vi "drive.vi"   [LabVIEW 2018]
uses:
  drive.ctl
  <vilib>/Rock Robotics/WPI/Utilities/WPI_GetSetVariantRefNum.vi
types:
  T1 = typedef "WPI_RobotDriveDevRef.ctl" = cluster{"DevStatus":errorcluster, "Motors[]":T2[], "Square Inputs":bool, "Max Output":dbl}
  T2 = typedef "WPI_MotorControlDeviceRef.ctl" = cluster{"DeviceStatus":errorcluster, "Type":T3, "PWM":cluster{"PWM Channel":T4, "DeadBand":T5}, "CAN":cluster{"Device Number":u8, "SetOutput VI Ref":variant, "GetOutput VI Ref":variant, "Enable VI Ref":variant, "Disable VI Ref":variant, "Data":variant}, "Invert":bool, "DIO PWM":cluster{"PWM \"Enable\" Channel":T4, "DIOChannel":T6, "PWM Rate":dbl}}
  T3 = typedef "WPI_MotorControlType.ctl" = enum16{"PWM", "CAN", "DIO PWM"}
  T4 = typedef "FPGA_DIOPWMChannel.ctl" = enum8{"PWM 0", "PWM 1", "PWM 2", "PWM 3", "PWM 4", "PWM 5", "PWM 6", "PWM 7", "PWM 8", "PWM 9", "PWM MXP 0", "PWM MXP 1", "PWM MXP 2", "PWM MXP 3", "PWM MXP 4", "PWM MXP 5", "PWM MXP 6", "PWM MXP 7", "PWM MXP 8", "PWM MXP 9", "Invalid"}
  T5 = typedef "WPI_PWMDeadband.ctl" = cluster{"Name":string, "maxPositivePwm":i32, "minPositivePwm":i32, "centerPwm":i32, "maxNegativePwm":i32, "minNegativePwm":i32, "angularRange":u16}
  T6 = typedef "FPGA_DIOChannel.ctl" = enum8{"DIO 0", "DIO 1", "DIO 2", "DIO 3", "DIO 4", "DIO 5", "DIO 6", "DIO 7", "DIO 8", "DIO 9", "DIO MXP 0", "DIO MXP 1", "DIO MXP 2", "DIO MXP 3", "DIO MXP 4", "DIO MXP 5", "DIO MXP 6", "DIO MXP 7", "DIO MXP 8", "DIO MXP 9", "DIO MXP 10", "DIO MXP 11", "DIO MXP 12", "DIO MXP 13", "DIO MXP 14", "DIO MXP 15", "SPI Port CS1", "SPI Port CS2", "SPI Port CS3", "SPI Port MISO", "SPI Port MOSI", "Invalid"}
  T7 = typedef "drive.ctl" = enum16{"noDrive", "Manual", "ManualWithPID"}
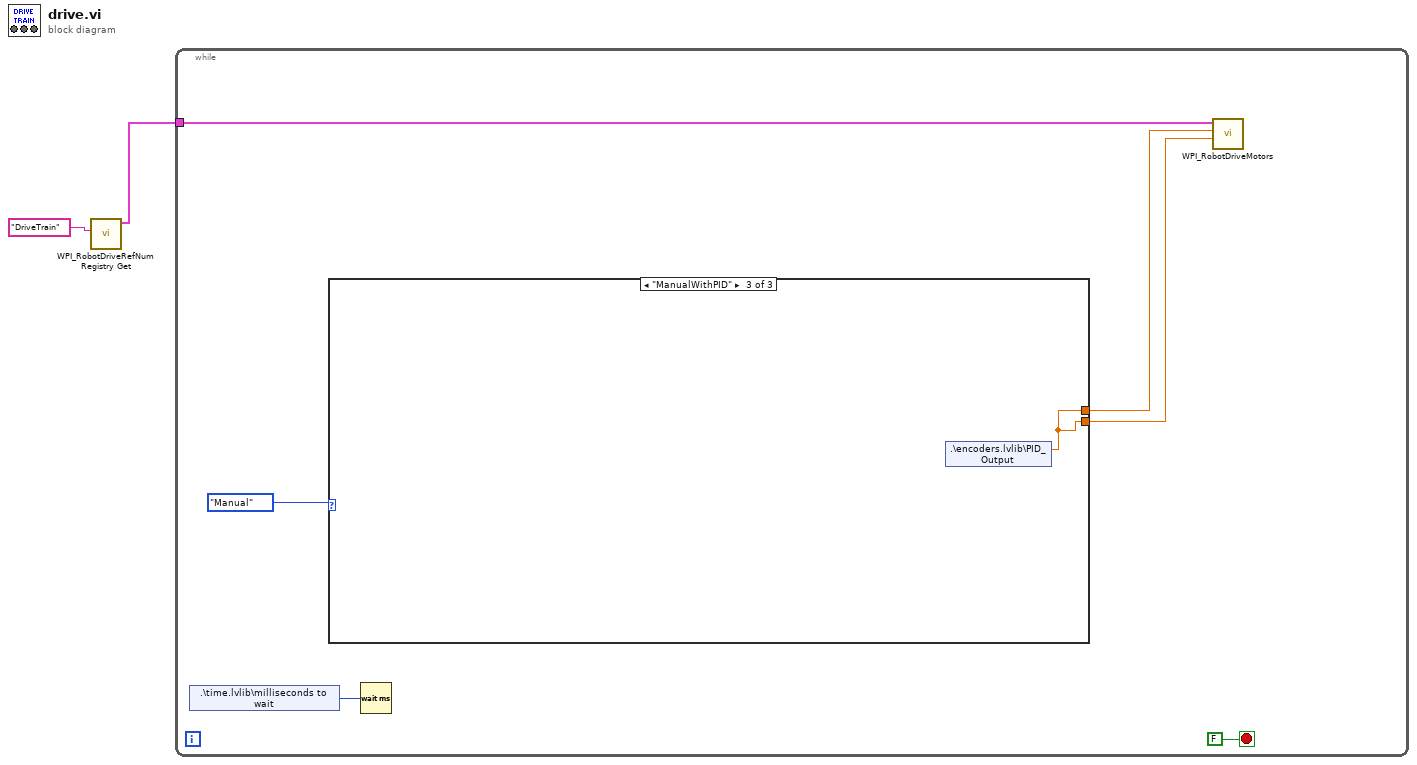
[diagram p0: block diagram]
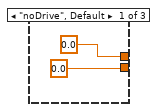
[diagram p2: hidden frame]
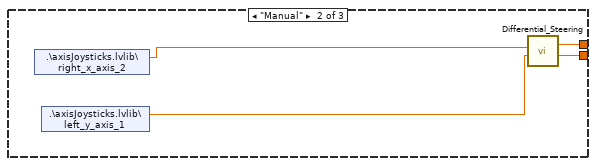
[diagram p3: hidden frame]
diagram:
  n1 = call <vilib>:"WPI_RobotDriveRefNum Registry Get.vi"("refnum name"="DriveTrain") -> ("RobotDriveDevRef"=w1:T1)  [unwired: 9 in, 1 out]
  n2 = while {
    tunnel: w1 -> [w6]
    stop <- FALSE stop-if-true
    n3 = shared-variable ".\\time.lvlib\\milliseconds to wait"() -> (w8:u32)  [unwired: 1 in, 1 out]
    n4 = case shown="\"ManualWithPID\"" drive."Manual" {
      tunnel: [0.0 ("Right") w12 w15] -> w4
      tunnel: [0.0 ("Left") w11 w15] -> w3
      frame "noDrive", Default {
      }
      frame "Manual" {
        n5 = shared-variable ".\\axisJoysticks.lvlib\\right_x_axis_2"() -> (w14:dbl)  [unwired: 1 in, 1 out]
        n6 = shared-variable ".\\axisJoysticks.lvlib\\left_y_axis_1"() -> (w13:dbl)  [unwired: 1 in, 1 out]
        n7 = call <userlib>:"Differential_Steering.vi"("Steer"=w13, "Base"=w14) -> ("Right"=w12:dbl, "Left"=w11:dbl)  [unwired: 4 in]
      }
      frame "ManualWithPID" {
        n8 = shared-variable ".\\encoders.lvlib\\PID_Output"() -> (w15:dbl)  [unwired: 1 in, 1 out]
      }
    }
    n9 = Wait (ms)(milliseconds to wait=w8) -> ()  [unwired: 1 out]
    n10 = call <vilib>:"WPI_RobotDriveMotors.vi"("RightSpeed"=w4, "LeftSpeed"=w3, "RobotDriveDevRef"=w6) -> ()  [unwired: 6 in, 3 out]
  }
